vi "Destroy.vi"(0 "reference in":refnum<class "Parent.lvclass">, 5 "error in (no error)":errorcluster) -> (14 "reference out":refnum<class "Parent.lvclass">, 19 "error out":errorcluster)   [LabVIEW 2019, in "Parent.lvclass"]
uses:
  Parent.lvclass
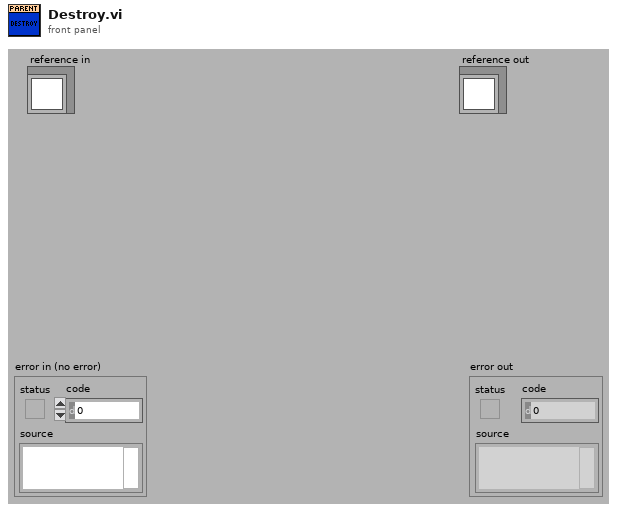
[diagram p1: front panel]
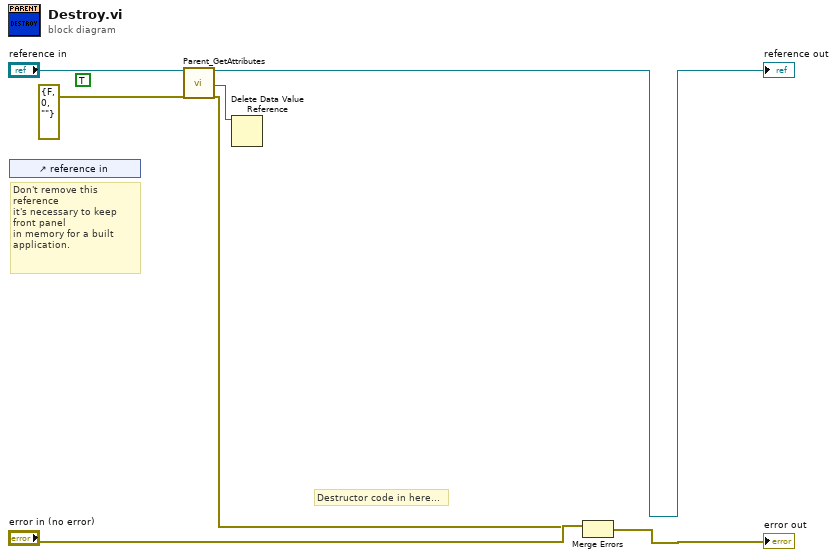
[diagram p0: block diagram]
diagram:
  (unwired) TRUE ("Simple Info")
  # "Don't remove this reference\nit's necessary to keep front panel\nin memory for a built application."
  # "Destructor code in here..."
  n1 = control-ref of="reference in"() -> ()  [unwired: 1 out]
  n2 = call "Parent_GetAttributes.vi"("reference in"="reference in", "error in (no error)"=errorcluster {"status"=FALSE, "code"=0, "source"=""}) -> ("reference out"=→"reference out":refnum<class "Parent.lvclass">, "DataRef"=w1:refnum<data-value>, "error out"=w5:errorcluster)  [unwired: 14 in, 1 out]
  n3 = Delete Data Value Reference(data value reference=w1) -> ()  [unwired: 1 in, 2 out]
  n4 = Merge Errors("error in (no error)", w5) -> (→"error out":errorcluster)
